vi "Manual Save.vi"(0 "机种":string, 5 "Command":enum16{"Write", "Read"}(ring), 11 "error in (no error)":errorcluster caption="错误输入（无错误）", 12 "Top":cluster{"下边缘设置：":i32, "右边缘设置：":i32}, 14 "Bottom":cluster{"上边缘设置：":i32, "右边缘设置：":i32}) -> (6 "Top Read":cluster{"下边缘设置：":i32, "右边缘设置：":i32}, 10 "Bottom read":cluster{"上边缘设置：":i32, "右边缘设置：":i32}, 15 "error out":errorcluster caption="错误输出")   [LabVIEW 2016]
uses:
  <vilib>/Utility/config.llb/Read Key (U32).vi
  <vilib>/Utility/config.llb/Write Key (I32).vi
  <vilib>/Utility/config.llb/NI_LVConfig.lvlib
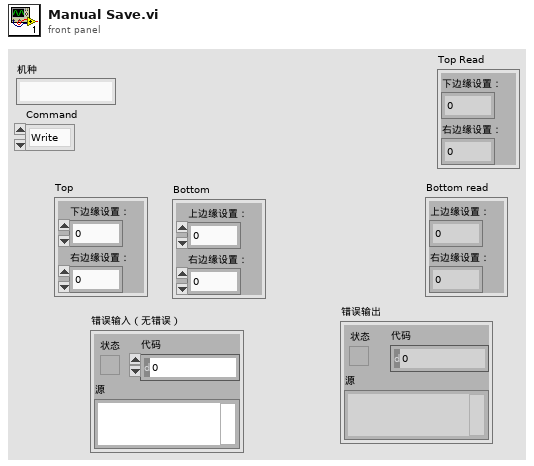
[diagram p1: front panel]
types:
  T1 = typedef "NI_LVConfig.lvlib/Config Data RefNum.ctl" = refnum<k1>
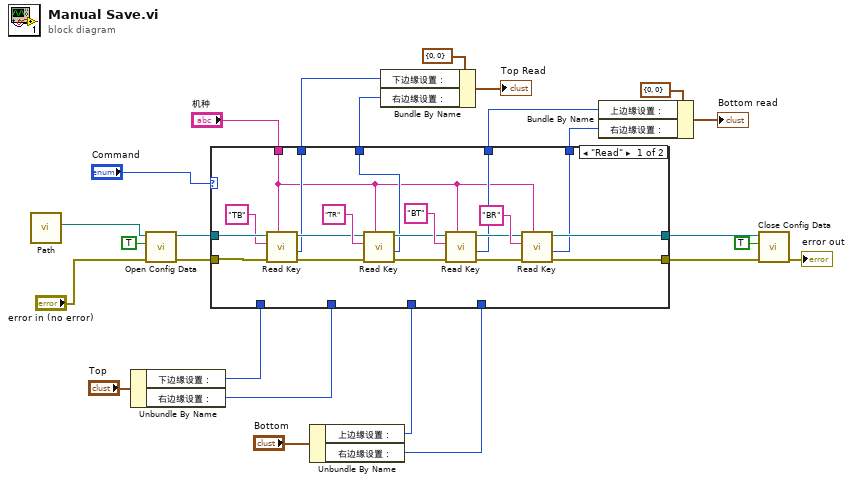
[diagram p0: block diagram]
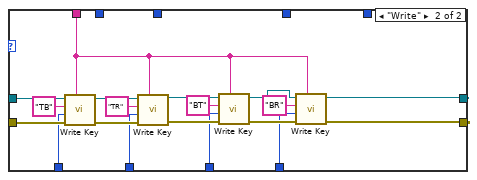
[diagram p2: hidden frame]
diagram:
  n1 = call "Path.vi"() -> ("ini"=w10:path)  [unwired: 11 in]
  n2 = Unbundle By Name("Top") -> ("下边缘设置："=w22:i32, "右边缘设置："=w21:i32)
  n3 = call <vilib>:"Open Config Data.vi"("error in (no error)"="error in (no error)", "create file if necessary (T)"=TRUE, "configuration file path"=w10) -> ("error out"=w24:errorcluster, "refnum"=w25:T1)  [unwired: 6 in, 1 out]
  n4 = Unbundle By Name("Bottom") -> ("上边缘设置："=w19:i32, "右边缘设置："=w18:i32)
  n5 = case shown="\"Read\"" "Command" {
    tunnel: w25 -> [w43 w63]
    tunnel: w24 -> [w44 w62]
    tunnel: w22 -> [_ w60]
    tunnel: w21 -> [_ w56]
    tunnel: w19 -> [_ w52]
    tunnel: w18 -> [_ w48]
    tunnel: "机种" -> [w26 w47]
    tunnel: [w38 w46] -> w16
    tunnel: [w37 w45] -> w15
    tunnel: [w30 _] -> w7
    tunnel: [w29 _] -> w6
    tunnel: [w28 _] -> w2
    tunnel: [w27 _] -> w1
    frame "Read" {
      n6 = call-poly <vilib>:"Read Key.vi"("section"=w26, "error in (no error)"=w44, "key"="TB", "refnum"=w43) -> ("error out"=w31:errorcluster, "value"=w30:u32, "refnum out"=w32:T1)  [unwired: 4 in, 1 out]
      n7 = call-poly <vilib>:"Read Key.vi"("section"=w26, "error in (no error)"=w31, "key"="TR", "refnum"=w32) -> ("error out"=w33:errorcluster, "value"=w29:u32, "refnum out"=w34:T1)  [unwired: 4 in, 1 out]
      n8 = call-poly <vilib>:"Read Key.vi"("section"=w26, "error in (no error)"=w33, "key"="BT", "refnum"=w34) -> ("error out"=w35:errorcluster, "value"=w28:u32, "refnum out"=w36:T1)  [unwired: 4 in, 1 out]
      n9 = call-poly <vilib>:"Read Key.vi"("section"=w26, "error in (no error)"=w35, "key"="BR", "refnum"=w36) -> ("error out"=w37:errorcluster, "value"=w27:u32, "refnum out"=w38:T1)  [unwired: 4 in, 1 out]
    }
    frame "Write" {
      n10 = call-poly <vilib>:"Write Key.vi"("section"=w47, "error in (no error)"=w62, "value"=w60, "key"="TB", "refnum"=w63) -> ("error out"=w57:errorcluster, "refnum out"=w58:T1)  [unwired: 4 in, 1 out]
      n11 = call-poly <vilib>:"Write Key.vi"("section"=w47, "error in (no error)"=w57, "value"=w56, "key"="TR", "refnum"=w58) -> ("error out"=w53:errorcluster, "refnum out"=w54:T1)  [unwired: 4 in, 1 out]
      n12 = call-poly <vilib>:"Write Key.vi"("section"=w47, "error in (no error)"=w53, "value"=w52, "key"="BT", "refnum"=w54) -> ("error out"=w49:errorcluster, "refnum out"=w50:T1)  [unwired: 4 in, 1 out]
      n13 = call-poly <vilib>:"Write Key.vi"("section"=w47, "error in (no error)"=w49, "value"=w48, "key"="BR", "refnum"=w50) -> ("error out"=w45:errorcluster, "refnum out"=w46:T1)  [unwired: 4 in, 1 out]
    }
  }
  n14 = Bundle By Name(cluster=cluster{"下边缘设置：":i32, "右边缘设置：":i32} {"下边缘设置："=0, "右边缘设置："=0} ("Top Read"), "下边缘设置："=w7, "右边缘设置："=w6) -> (→"Top Read":cluster{"下边缘设置：":i32, "右边缘设置：":i32})
  n15 = Bundle By Name(cluster=cluster{"上边缘设置：":i32, "右边缘设置：":i32} {"上边缘设置："=0, "右边缘设置："=0} ("Bottom read"), "上边缘设置："=w2, "右边缘设置："=w1) -> (→"Bottom read":cluster{"上边缘设置：":i32, "右边缘设置：":i32})
  n16 = call <vilib>:"Close Config Data.vi"("error in (no error)"=w15, "write file if changed (T)"=TRUE, "refnum"=w16) -> ("error out"=→"error out":errorcluster)  [unwired: 7 in, 1 out]
